vi "FL30XX_simple.vi"() -> ()   [LabVIEW 2015]
uses:
  board.vis/Globals.vi
  board.vis/ESLSCDLL.lvlib
panel:
  in  "value black":u32
  in  "value white":u32=65535
  in  "show greyscale viewer":bool
  in  "Live view":enum32{"off", "current sample", "fixed sample"}(radio)
  in  "abort":bool
  in  "no.of blocks (nob)":u32=1 min=1
  in  "no.of samples (nos)":u32=1000 min=2
  in  "continuous":bool
  in  "exit":bool
  out "Signal Cam 2":u16[](graph)
  out "Measure ON":bool
  in  "block":u32(slide)=1 min=1 max=1 scale=0.9..1.0
  out "Signal Cam1":u16[](graph)=[0, 0, 0, 1, 0, 46, 0, 0, 0, 0, 0, 381, 404, 443, 578, 571, 486, 447, 419, 401, 394, 388, 388, 395, 397, 408, 404, 397, 378, 403, 397, 394, 392, 403, 406, 406, 408, 385, 385, 387, 397, 392, 392, 406, 399, 392, 395, 394, 404, 392, 399, 399, 401, 388, 383, 381, 392, 411, 399, 394, 397, 383, 399, 390, 397, 385, 380, 383, 381, 395, 395, 387, 403, 394, 392, 392, 390, 394, 406, 390, 388, 401, 387, 378, 394, 397, 385, 394, 397, 406, 404, 387, 385, 394, 388, 413, 592, 740, 589, 454, 404, 392, 401, 417, 411, 394, 392, 381, 380, 383, 392, 406, 399, 383, 390, 392, 399, 387, 404, 394, 394, 394, 388, 387, 397, 404, 415, 394, 385, 392, 399, 387, 390, 387, 397, 395, 383, 392, 392, 353, 362, 369, 364, 356, 371, 364, 362, 365, 356, 353, 365, 374, 367, 381, 369, 374, 358, 383, 388, 395, 411, 933, 1697, 1195, 647, 426, 383, 372, 374, 362, 372, 380, 380, 371, 372, 376, 372, 365, 376, 371, 374, 362, 358, 364, 358, 376, 369, 362, 364, 364, 371, 374, 362, 356, 351, 358, 351, 364, 369, 360, 369, 364, 362, 364, 358, 364, 372, 362, 364, 362, 351, 356, 371, 365, 362, 360, 367, 376, 372, 360, 356, 364, 356, 358, 380, 369, 364, 376, 360, 358, 358, 372, 369, 365, 360, 353, 349, 364, 369, 378, 365, 367, 365, 367, 372, 367, 372, 365, 369, 369, 355, 358, 374, 374, 387, 371, 355, 365, 378, 362, 353, 365, 362, 360, 353, 358, 358, 362, 364, 372, 365, 362, 378, 369, 365, 369, 365, 367, 364, 372, 371, 376, 372, 365, 364, 369, 372, 365, 372, 395, 385, 381, 390, 369, 367, 371, 380, 367, 387, 392, 387, 385, 390, 395, 404, 403, 436, 468, 507, 578, 818, 4075, 10655, 8844, 5265, 2006, 853, 567, 500, 456, 433, 403, 399, 397, 376, 392, 383, 378, 388, 387, 378, 376, 369, 376, 381, 358, 367, 372, 364, 364, 371, 372, 372, 369, 367, 378, 372, 360, 356, 362, 358, 360, 378, 372, 374, 372, 364, 362, 371, 371, 372, 376, 372, 364, 355, 360, 360, 371, 374, 362, 364, 360, 362, 355, 371, 362, 365, 365, 360, 360, 364, 372, 374, 369, 356, 358, 367, 358, 360, 364, 367, 374, 392, 896, 896, 1383, 986, 610, 424, 371, 369, 353, 351, 358, 349, 348, 348, 353, 356, 353, 358, 355, 344, 356, 353, 360, 344, 351, 358, 356, 360, 351, 349, 344, 355, 353, 355, 360, 360, 349, 349, 349, 356, 349, 353, 353, 355, 346, 346, 351, 362, 367, 360, 353, 353, 348, 360, 353, 353, 339, 330, 342, 335, 344, 349, 348, 355, 353, 351, 463, 481, 442, 410, 431, 513, 461, 419, 376, 353, 351, 348, 349, 351, 351, 349, 339, 333, 342, 342, 344, 355, 348, 349, 348, 349, 340, 348, 355, 356, 342, 339, 330, 340, 346, 372, 376, 369, 351, 358, 348, 349, 339, 353, 349, 342, 344, 333, 349, 339, 349, 360, 346, 337, 340, 353, 340, 342, 342, 351, 355, 340, 349, 349, 305, 321, 312, 317, 309, 312, 314, 312, 321, 310, 316, 307, 316, 314, 317, 321, 316, 312, 321, 316, 310, 307, 321, 328, 317, 323, 314, 310, 312, 316, 314, 316, 314, 319, 316, 312, 312, 321, 317, 355, 351, 372, 387, 369, 346, 333, 328, 321, 309, 319, 314, 314, 316, 309, 305, 307, 307, 305, 309, 309, 310, 310, 310, 310, 317, 310, 307, 314, 310, 309, 309, 309, 305, 314, 309, 314, 305, 312, 314, 305, 301, 303, 314, 314, 301, 310, 310, 312, 316, 301, 303, 301, 314, 312, 300, 303, 296, 298, 303, 307, 309, 309, 300, 312, 310, 314, 305, 310, 305, 309, 307, 303, 303, 310, 316, 312, 309, 307, 303, 309, 303, 307, 305, 314, 314, 303, 309, 309, 305, 307, 326, 314, 312, 321, 319, 310, 317, 316, 312, 312, 314, 316, 316, 321, 316, 309, 323, 319, 312, 316, 316, 319, 316, 319, 316, 309, 316, 316, 314, 312, 323, 321, 312, 314, 316, 321, 316, 310, 316, 314, 310, 312, 316, 321, 317, 319, 312, 316, 316, 319, 316, 321, 309, 305, 307, 301, 310, 316, 310, 323, 314, 310, 325, 317, 325, 319, 316, 316, 312, 310, 309, 312, 309, 310, 309, 305, 312, 309, 303, 303, 307, 312, 310, 314, 310, 310, 316, 307, 307, 309, 316, 310, 307, 309, 309, 310, 305, 312, 309, 312, 300, 310, 309, 309, 305, 314, 309, 312, 312, 309, 307, 312, 309, 314, 309, 305, 303, 314, 300, 303, 303, 310, 307, 301, 307, 307, 312, 326, 328, 321, 319, 330, 326, 325, 330, 346, 342, 351, 337, 333, 333, 332, 328, 321, 330, 328, 323, 323, 321, 328, 325, 328, 314, 332, 321, 325, 326, 323, 326, 326, 326, 328, 328, 325, 316, 321, 319, 321, 317, 317, 321, 321, 326, 323, 316, 325, 319, 325, 321, 328, 332, 326, 339, 323, 332, 333, 325, 333, 323, 312, 317, 314, 323, 325, 317, 317, 316, 319, 319, 321, 330, 369, 585, 651, 631, 573, 504, 484, 484, 456, 401, 378, 349, 340, 340, 332, 317, 314, 321, 319, 321, 316, 309, 310, 314, 321, 330, 330, 325, 328, 326, 330, 326, 330, 317, 319, 321, 316, 319, 314, 325, 325, 316, 314, 316, 319, 310, 310, 310, 317, 321, 307, 312, 312, 291, 298, 305, 300, 305, 305, 298, 300, 303, 307, 301, 296, 298, 300, 298, 303, 301, 296, 294, 301, 303, 303, 312, 314, 310, 310, 307, 298, 303, 309, 307, 303, 303, 298, 307, 307, 305, 312, 309, 312, 305, 307, 300, 305, 300, 303, 303, 293, 289, 293, 301, 300, 301, 298, 301, 314, 316, 312, 316, 333, 340, 337, 321, 326, 314, 309, 310, 310, 305, 296, 298, 293, 298, 296, 298, 296, 298, 296, 296, 300, 294, 293, 293, 296, 296, 303, 298, 298, 296, 296, 289, 296, 301, 305, 305, 296, 293, 294, 298, 294, 300, 298, 294, 300, 294, 298, 294, 291, 289, 293, 294, 296, 293, 294, 298, 0, 46]
  in  "start":bool
  in  "sample":u32(slide)=46 min=1 max=1000 scale=1.0..1000.0
  # "press cont to stop"
  # "Use exit button to quit!"
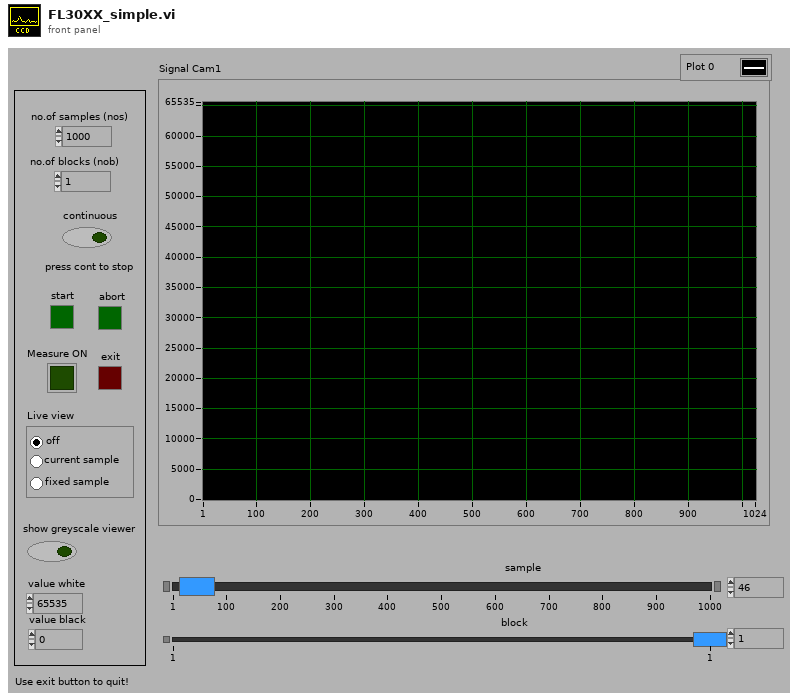
[diagram p1: front panel]
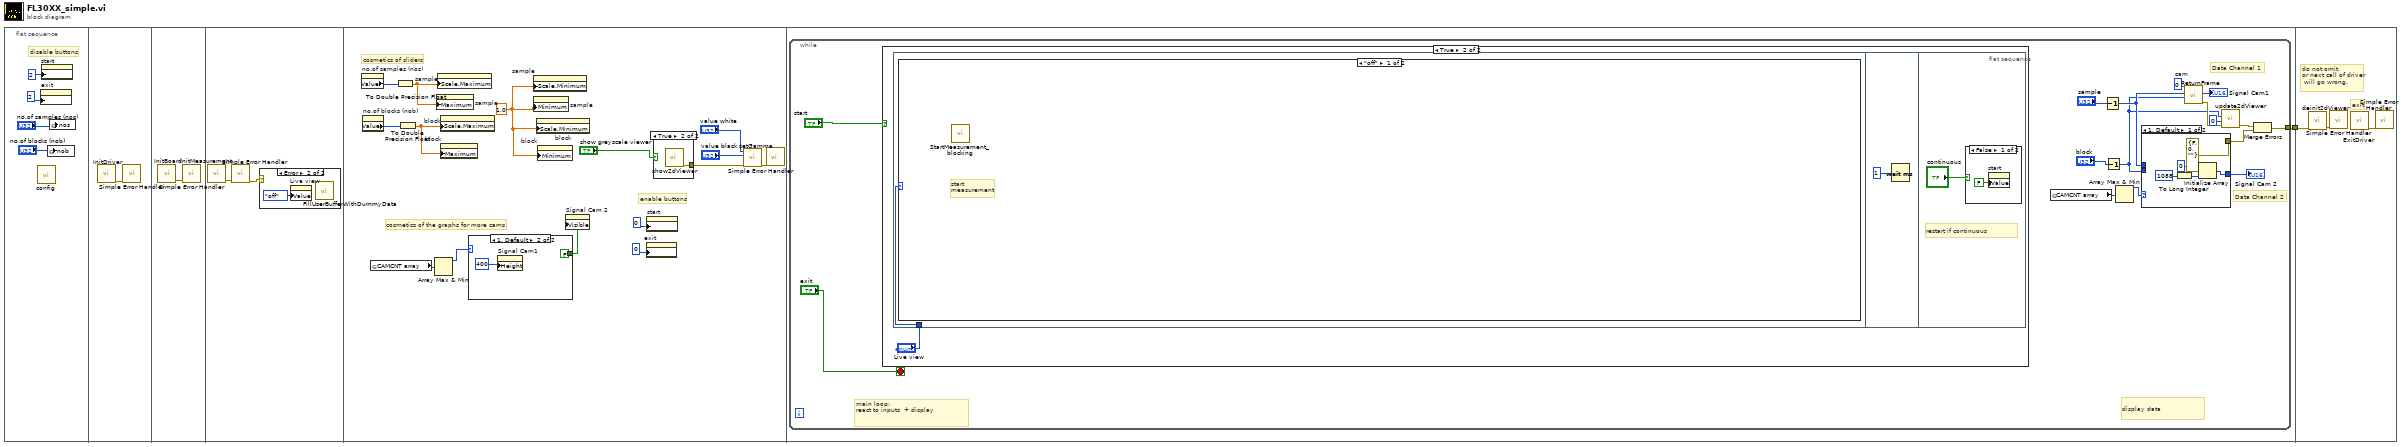
[diagram p0: block diagram]
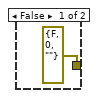
[diagram p3: hidden frame]
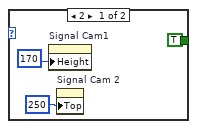
[diagram p4: hidden frame]
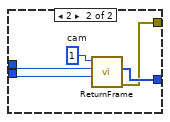
[diagram p5: hidden frame]
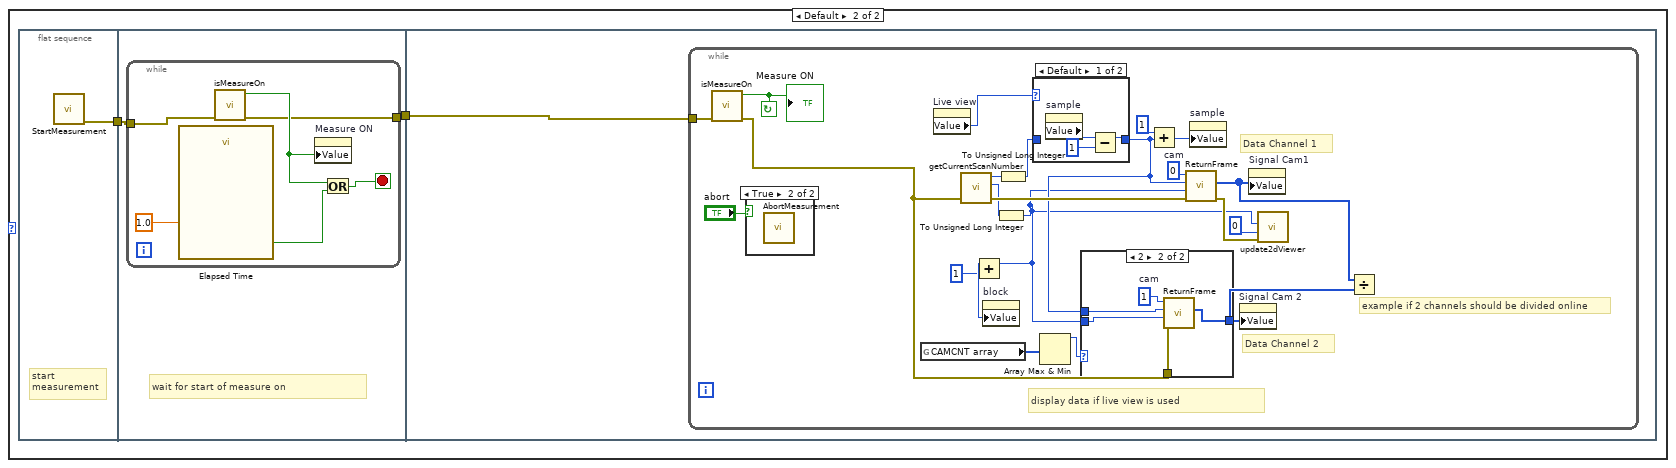
[diagram p7: hidden frame]
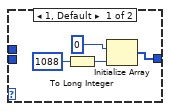
[diagram p9: hidden frame]
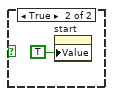
[diagram p11: hidden frame]
diagram:
  n1 = flat-sequence {
    tunnel: [w33] -> w1
    tunnel: w1 -> [w113]
    frame #0 {
      # "disable buttons"
      n2 = call "config.vi"() -> ()  [unwired: 12 in]
      n3 = property on="exit" class="Bool (strict)"("DisabledEnum"=u32 2) -> ()  [unwired: 2 in, 2 out]
      n4 = property on="start" class="Bool (strict)"("DisabledEnum"=u32 2) -> ()  [unwired: 2 in, 2 out]
      n5 = global write "Globals.vi" "nob"("no.of blocks (nob)") -> ()
      n6 = global write "Globals.vi" "nos"("no.of samples (nos)") -> ()
    }
    frame #1 {
      n7 = call "InitDriver.vi"() -> ("error out"=w6:errorcluster)  [unwired: 11 in]
      n8 = call <vilib>:"Simple Error Handler.vi"("error in (no error)"=w6) -> ()  [unwired: 4 in, 5 out]
    }
    frame #2 {
      n9 = call "InitBoard.vi"() -> ("error out"=w7:errorcluster)  [unwired: 10 in]
      n10 = call <vilib>:"Simple Error Handler.vi"("error in (no error)"=w7) -> ()  [unwired: 4 in, 5 out]
    }
    frame #3 {
      n11 = call "InitMeasurement.vi"() -> ("error out"=w8:errorcluster)  [unwired: 11 in]
      n12 = call <vilib>:"Simple Error Handler.vi"("error in (no error)"=w8) -> ("error out"=w9:errorcluster)  [unwired: 4 in, 4 out]
      n13 = case shown="Error" w9 {
        frame No Error {
        }
        frame Error {
          n14 = property on="Live view" class="RadioBtnsControl (strict)"("Value"=enum32{"off", "current sample", "fixed sample"}."off" ("Live view")) -> ()  [unwired: 2 in, 2 out]
          n15 = call "FillUserBufferWithDummyData.vi"() -> ()  [unwired: 11 in, 1 out]
        }
      }
    }
    frame #4 {
      w18 = 1.0 ("Scale.Range:Minimum")
      # "enable buttons"
      # "cosmetics of sliders"
      # "cosmetics of the graphs for more cams"
      n16 = property on="no.of samples (nos)" class="DigNum (strict)"() -> ("Value"=w22:u32)  [unwired: 2 in, 2 out]
      n17 = property on="no.of blocks (nob)" class="DigNum (strict)"() -> ("Value"=w21:u32)  [unwired: 2 in, 2 out]
      n18 = global read "Globals.vi" "CAMCNT array"() -> (w13:u32[])
      n19 = To Double Precision Float(number=w22) -> (double precision float=w19:dbl)
      n20 = To Double Precision Float(number=w21) -> (double precision float=w20:dbl)
      n21 = Array Max & Min(array=w13) -> (max value=w12:u32)  [unwired: 3 out]
      n22 = property on="sample" class="Slide (strict)"("Maximum"=w19) -> ()  [unwired: 2 in, 2 out]
      n23 = property on="sample" class="Slide (strict)"("Scale.Maximum"=w19) -> ()  [unwired: 2 in, 2 out]
      n24 = property on="block" class="Slide (strict)"("Scale.Maximum"=w20) -> ()  [unwired: 2 in, 2 out]
      n25 = property on="block" class="Slide (strict)"("Maximum"=w20) -> ()  [unwired: 2 in, 2 out]
      n26 = case shown="1, Default" w12 {
        tunnel: [TRUE FALSE] -> w25
        frame 2 {
          n27 = property on="Signal Cam1" class="WFGraph (strict)"("Height"=u32 170) -> ()  [unwired: 2 in, 2 out]
          n28 = property on="Signal Cam 2" class="WFGraph (strict)"("Top"=250) -> ()  [unwired: 2 in, 2 out]
        }
        frame 1, Default {
          n29 = property on="Signal Cam1" class="WFGraph (strict)"("Height"=u32 400) -> ()  [unwired: 2 in, 2 out]
        }
      }
      n30 = property on="sample" class="Slide (strict)"("Minimum"=w18) -> ()  [unwired: 2 in, 2 out]
      n31 = property on="sample" class="Slide (strict)"("Scale.Minimum"=w18) -> ()  [unwired: 2 in, 2 out]
      n32 = property on="block" class="Slide (strict)"("Scale.Minimum"=w18) -> ()  [unwired: 2 in, 2 out]
      n33 = property on="block" class="Slide (strict)"("Minimum"=w18) -> ()  [unwired: 2 in, 2 out]
      n34 = property on="Signal Cam 2" class="WFGraph (strict)"("Visible"=w25) -> ()  [unwired: 2 in, 2 out]
      n35 = property on="exit" class="Bool (strict)"("DisabledEnum"=u32 0) -> ()  [unwired: 2 in, 2 out]
      n36 = property on="start" class="Bool (strict)"("DisabledEnum"=u32 0) -> ()  [unwired: 2 in, 2 out]
      n37 = case shown="True" "show greyscale viewer" {
        tunnel: [errorcluster {"status"=FALSE, "code"=0, "source"=""} ("error out") w27] -> w16
        frame False {
        }
        frame True {
          n38 = call "show2dViewer.vi"() -> ("error out"=w27:errorcluster)  [unwired: 11 in]
        }
      }
      n39 = call "setGamma.vi"("error in (no error)"=w16, "black"="value black", "white"="value white") -> ("error out"=w11:errorcluster)  [unwired: 8 in]
      n40 = call <vilib>:"Simple Error Handler.vi"("error in (no error)"=w11) -> ()  [unwired: 4 in, 5 out]
    }
    frame #5 {
      n41 = while {
        tunnel: [w44] -> w33
        stop <- "exit" stop-if-true
        w43 = u16 0  # cam
        # "Data Channel 2"
        # "Data Channel 1"
        # "main loop:\nreact to inputs  + display"
        # "display data"
        n42 = case shown="True" "start" {
          frame False {
          }
          frame True {
            n43 = flat-sequence {
              tunnel: "Live view" -> [w61]
              frame #0 {
                n44 = case shown="\"off\"" w61 {
                  frame "off" {
                    # "start\nmeasurement"
                    n45 = call "StartMeasurement_blocking.vi"() -> ()  [unwired: 11 in, 1 out]
                  }
                  frame Default {
                    n46 = flat-sequence {
                      tunnel: [w64] -> w63
                      tunnel: w63 -> [w66]
                      tunnel: [w65] -> w62
                      tunnel: w62 -> [w73]
                      frame #0 {
                        # "start\nmeasurement"
                        n47 = call "StartMeasurement.vi"() -> ("error out"=w64:errorcluster)  [unwired: 11 in]
                      }
                      frame #1 {
                        # "wait for start of measure on"
                        n48 = while {
                          tunnel: w66 -> [w68]
                          tunnel: [w67] -> w65
                          stop <- w71 stop-if-true
                          n49 = call "Elapsed Time"("Time Target (s)"=1.0) -> ("Time has Elapsed"=w70:bool)  [unwired: 11 in, 7 out]
                          n50 = call "isMeasureOn.vi"("error in (no error)"=w68) -> ("error out"=w67:errorcluster, "Measure On 1"=w69:bool)  [unwired: 8 in, 1 out]
                          n51 = property on="Measure ON" class="Bool (strict)"("Value"=w69) -> ()  [unwired: 2 in, 2 out]
                          n52 = Or(x=w69, y=w70) -> (x .or. y?=w71:bool)
                        }
                      }
                      frame #2 {
                        n53 = while {
                          tunnel: w73 -> [w93]
                          stop <- w94 continue-if-true
                          w90 = u16 0  # cam
                          # "example if 2 channels should be divided online"
                          # "Data Channel 2"
                          # "Data Channel 1"
                          # "display data if live view is used"
                          n54 = call "isMeasureOn.vi"("error in (no error)"=w93) -> ("error out"=w91:errorcluster, "Measure On 1"=w94:bool)  [unwired: 8 in, 1 out]
                          "Measure ON" <- w94
                          n55 = case shown="True" "abort" {
                            frame False {
                            }
                            frame True {
                              n56 = call "AbortMeasurement.vi"() -> ()  [unwired: 10 in, 1 out]
                            }
                          }
                          n57 = global read "Globals.vi" "CAMCNT array"() -> (w75:u32[])
                          n58 = property on="Live view" class="RadioBtnsControl (strict)"() -> ("Value"=w83:enum32{"off", "current sample", "fixed sample"})  [unwired: 2 in, 2 out]
                          n59 = call "getCurrentScanNumber.vi"() -> ("block"=w88:i64, "sample"=w89:i64)  [unwired: 9 in, 1 out]
                          n60 = To Unsigned Long Integer(number=w88) -> (unsigned 32bit integer=w78:u32)
                          n61 = Add(x=w78, y=u32 1) -> (x+y=w85:u32)
                          n62 = property on="block" class="Slide (strict)"("Value"=w85) -> ()  [unwired: 2 in, 2 out]
                          n63 = To Unsigned Long Integer(number=w89) -> (unsigned 32bit integer=w82:u32)
                          n64 = case shown="Default" w83 {
                            tunnel: w82 -> [_ w98]
                            tunnel: [w96 w98] -> w81
                            frame Default {
                              n65 = property on="sample" class="Slide (strict)"() -> ("Value"=w97:u32)  [unwired: 2 in, 2 out]
                              n66 = Subtract(x=w97, y=u32 1) -> (x-y=w96:u32)
                            }
                            frame "current sample" {
                            }
                          }
                          n67 = Array Max & Min(array=w75) -> (max value=w74:u32)  [unwired: 3 out]
                          n68 = case shown="2" w74 {
                            tunnel: [w99 w107] -> w76
                            tunnel: w91 -> [_ w106]
                            tunnel: w81 -> [_ w104]
                            tunnel: w78 -> [_ w103]
                            frame 1, Default {
                              n69 = To Long Integer(number=u16 1088) -> (32bit integer=w100:i32)
                              n70 = Initialize Array(u16 0, w100) -> (w99:u16[])
                            }
                            frame 2 {
                              w105 = u16 1  # cam
                              n71 = call "ReturnFrame.vi"("error in (no error)"=w106, "block"=w103, "sample"=w104, "camera"=w105) -> ("Data Values Out 1"=w107:u16[])  [unwired: 5 in, 2 out]
                            }
                          }
                          n72 = Add(x=u32 1, y=w81) -> (x+y=w87:u32)
                          n73 = call "ReturnFrame.vi"("error in (no error)"=w91, "block"=w78, "sample"=w81, "camera"=w90) -> ("error out"=w79:errorcluster, "Data Values Out 1"=w77:u16[])  [unwired: 5 in, 1 out]
                          n74 = property on="sample" class="Slide (strict)"("Value"=w87) -> ()  [unwired: 2 in, 2 out]
                          n75 = property on="Signal Cam 2" class="WFGraph (strict)"("Value"=w76) -> ()  [unwired: 2 in, 2 out]
                          n76 = property on="Signal Cam1" class="WFGraph (strict)"("Value"=w77) -> ()  [unwired: 2 in, 2 out]
                          n77 = call "update2dViewer.vi"("error in (no error)"=w79, "camera"=u16 0 ("cam"), "block"=w78) -> ()  [unwired: 8 in, 1 out]
                          n78 = Divide(x=w77, y=w76) -> ()  [unwired: 1 out]
                        }
                      }
                    }
                  }
                }
              }
              frame #1 {
                n79 = Wait (ms)(milliseconds to wait=u32 1) -> ()  [unwired: 1 out]
              }
              frame #2 {
                # "restart if continuous"
                n80 = case shown="False" "continuous" {
                  frame False {
                    n81 = property on="start" class="Bool (strict)"("Value"=FALSE ("start")) -> ()  [unwired: 2 in, 2 out]
                  }
                  frame True {
                    n82 = property on="start" class="Bool (strict)"("Value"=TRUE ("start")) -> ()  [unwired: 2 in, 2 out]
                  }
                }
              }
            }
          }
        }
        n83 = global read "Globals.vi" "CAMCNT array"() -> (w37:u32[])
        n84 = Decrement(x="sample") -> (x-1=w47:u32)
        n85 = Decrement(x="block") -> (x-1=w38:u32)
        n86 = Array Max & Min(array=w37) -> (max value=w36:u32)  [unwired: 3 out]
        n87 = case shown="1, Default" w36 {
          tunnel: w38 -> [_ w59]
          tunnel: w47 -> [_ w58]
          tunnel: [w51 w57] -> w48
          tunnel: [errorcluster {"status"=FALSE, "code"=0, "source"=""} ("error out") w56] -> w45
          frame 1, Default {
            n88 = To Long Integer(number=u16 1088) -> (32bit integer=w52:i32)
            n89 = Initialize Array(u16 0, w52) -> (w51:u16[])
          }
          frame 2 {
            w55 = u16 1  # cam
            n90 = call "ReturnFrame.vi"("block"=w59, "sample"=w58, "camera"=w55) -> ("error out"=w56:errorcluster, "Data Values Out 1"=w57:u16[])  [unwired: 6 in, 1 out]
          }
        }
        "Signal Cam 2" <- w48
        n91 = call "ReturnFrame.vi"("block"=w38, "sample"=w47, "camera"=w43) -> ("error out"=w41:errorcluster, "Data Values Out 1"=→"Signal Cam1":u16[])  [unwired: 6 in, 1 out]
        n92 = call "update2dViewer.vi"("error in (no error)"=w41, "camera"=u16 0 ("cam"), "block"=w38) -> ("error out"=w40:errorcluster)  [unwired: 8 in]
        n93 = Merge Errors(w40, w45) -> (w44:errorcluster)
      }
    }
    frame #6 {
      # "exit"
      # "do not omit, \nor next call of driver\n will go wrong."
      n94 = call "deinit2dViewer.vi"("error in (no error)"=w113) -> ("error out"=w112:errorcluster)  [unwired: 10 in]
      n95 = call <vilib>:"Simple Error Handler.vi"("error in (no error)"=w112) -> ()  [unwired: 4 in, 5 out]
      n96 = call "ExitDriver.vi"() -> ("error out"=w114:errorcluster)  [unwired: 11 in]
      n97 = call <vilib>:"Simple Error Handler.vi"("error in (no error)"=w114) -> ()  [unwired: 4 in, 5 out]
    }
  }
